vi "堆栈（Variant）.vi"(6 "堆栈长度":i32=256, 8 "error in (no error)":errorcluster caption="错误输入（无错误）", 9 "堆栈操作":T1, 11 "入栈元素(str)":variant) -> (0 "error out":errorcluster caption="错误输出", 1 "已用堆栈长度":i32, 3 "出栈元素":variant, 4 "堆栈空":bool, 5 "堆栈满":bool)   [LabVIEW 2012, in "Array Stack.lvlib"]
uses:
  Array Stack.lvlib
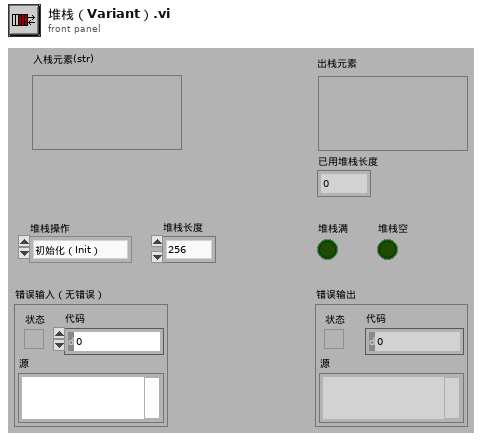
[diagram p1: front panel]
types:
  T1 = typedef "Array Stack.lvlib/堆栈操作.ctl" = enum16{"初始化（Init）", "进栈（Push）", "出栈（Pop）", "状态（Status)", "释放"}
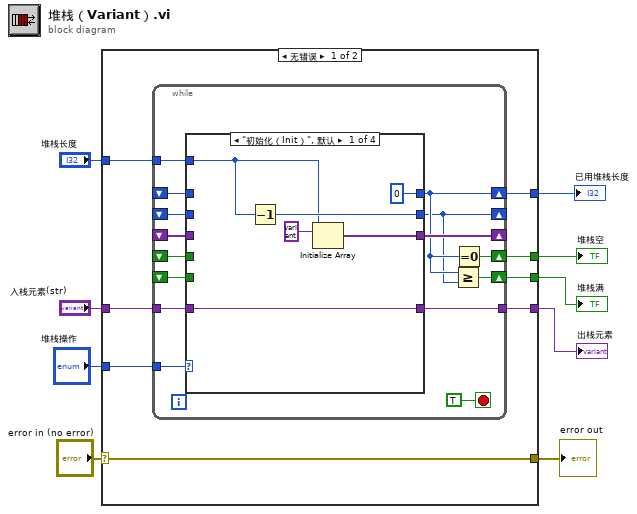
[diagram p0: block diagram]
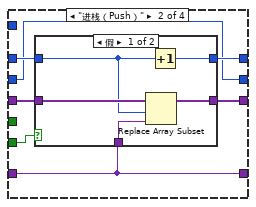
[diagram p2: hidden frame]
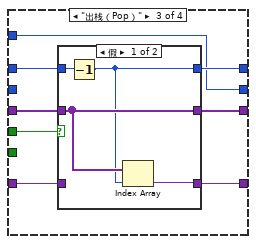
[diagram p4: hidden frame]
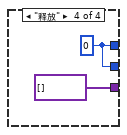
[diagram p6: hidden frame]
diagram:
  n1 = case shown="无错误" "error in (no error)" {
    selector: "error in (no error)" -> [w17 w70]
    tunnel: [w17 w70] -> w8
    tunnel: "堆栈操作" -> [w16 _]
    tunnel: "入栈元素(str)" -> [w15 _]
    tunnel: [w14 _] -> w5
    tunnel: [w10 _] -> w4
    tunnel: "堆栈长度" -> [w11 _]
    tunnel: [w13 _] -> w1
    tunnel: [w12 _] -> w2
    frame No Error {
      n2 = while {
        tunnel: w16 -> [w32]
        tunnel: w15 -> [w31]
        tunnel: [w30] -> w14
        tunnel: w11 -> [w28]
        shift-right: [w29] -> _
        shift-left: _ -> [w25]
        shift-right: [w18] -> _
        shift-left: _ -> [w19]
        shift-right: [w22] -> w10
        shift-left: _ -> [w20]
        shift-right: [w24] -> w13
        shift-left: _ -> [w26]
        shift-right: [w23] -> w12
        shift-left: _ -> [w21]
        stop <- TRUE stop-if-true
        n3 = case shown="\"初始化（Init）\", 默认" w32 {
          tunnel: w31 -> [w38 w45 w54 _]
          tunnel: [w38 w45 w56 _] -> w30
          tunnel: [0 ("堆栈长度") w43 w58 w69] -> w22
          tunnel: [w36 w41 w55 variant[] []] -> w29
          tunnel: w28 -> [w34 _ w53 _]
          tunnel: w20 -> [_ w44 w59 _]
          tunnel: w19 -> [_ w39 _ _]
          tunnel: w26 -> [_ w40 _ _]
          tunnel: w25 -> [_ w42 w57 _]
          tunnel: w21 -> [_ _ w60 _]
          tunnel: [w35 w39 w53 w69] -> w18
          frame "初始化（Init）", Default {
            n4 = Decrement(x=w34) -> (x-1=w35:i32)
            n5 = Initialize Array(variant ("入栈元素(str)"), w34) -> (w36:variant[])
          }
          frame "进栈（Push）" {
            n6 = case shown="假" w40 {
              tunnel: w45 -> [w49 _]
              tunnel: w44 -> [w46 w52]
              tunnel: [w50 w52] -> w43
              tunnel: w42 -> [w47 w51]
              tunnel: [w48 w51] -> w41
              frame False {
                n7 = Replace Array Subset(array=w47, new element=w49, index=w46) -> (w48:variant[])
                n8 = Increment(x=w46) -> (x+1=w50:i32)
              }
              frame True {
              }
            }
          }
          frame "出栈（Pop）" {
            n9 = case shown="假" w60 {
              tunnel: w59 -> [w62 w65]
              tunnel: [w61 w65] -> w58
              tunnel: w57 -> [w63 w67]
              tunnel: [w64 w66] -> w56
              tunnel: [w63 w67] -> w55
              tunnel: w54 -> [_ w66]
              frame False {
                n10 = Decrement(x=w62) -> (x-1=w61:i32)
                n11 = Index Array(array=w63, index=w61) -> (element=w64:variant)
              }
              frame True {
              }
            }
          }
          frame "释放" {
            w69 = 0 ("堆栈长度")
          }
        }
        n12 = Greater Or Equal?(x=w22, y=w18) -> (x >= y?=w24:bool)
        n13 = Equal To 0?(x=w22) -> (x = 0?=w23:bool)
      }
    }
    frame Error {
    }
  }
  "error out" <- w8
  "出栈元素" <- w5
  "已用堆栈长度" <- w4
  "堆栈满" <- w1
  "堆栈空" <- w2
